vi "Input Multiplexer to FFT (2 inputs)_I16.vi"(7 "Reset?":bool, 8 "Input Data Valid Array":bool[](array[boolean])=[FALSE, FALSE], 11 "Input Data":fxp<+/-,16,2>[](array[numeric])=[0.0, 0.0]) -> (0 "Output Data Valid Array":bool[](array[boolean]), 3 "Interchanged Data":fxp<+/-,16,2>[](array[numeric]) format="%.15g")   [LabVIEW 2011]
uses:
  <userlib>/FPGA Library/Code Development/Signal Processing/Input Multiplexer to FFT/2 Input MUX/Input Index(Type) 2 inputs.ctl
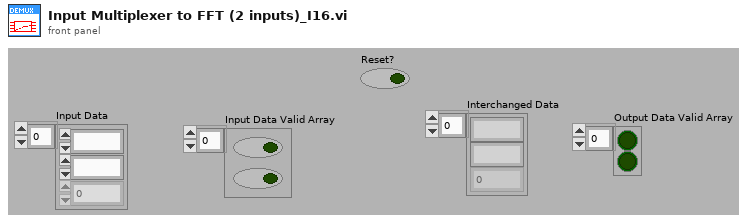
[diagram p1: front panel]
types:
  T1 = typedef "Input Index(Type) 2 inputs.ctl" = fxp<+,1,1>
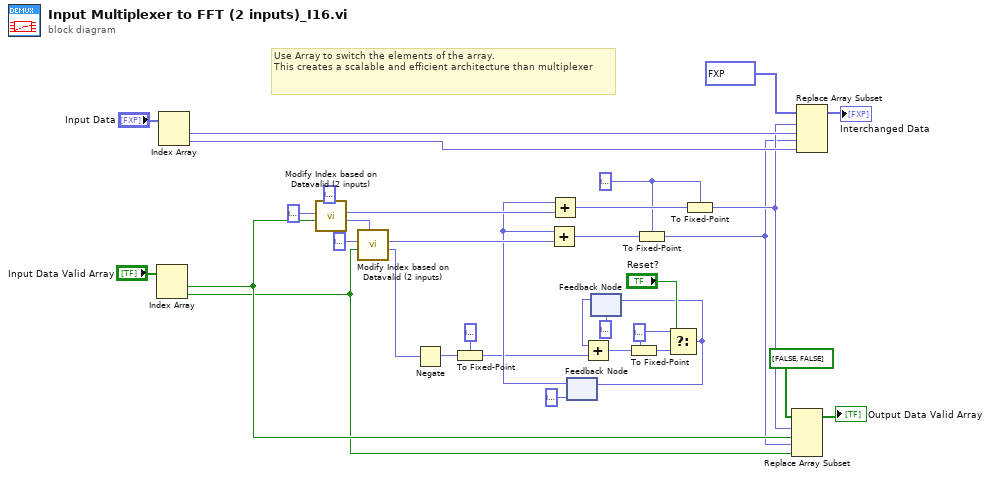
[diagram p0: block diagram]
diagram:
  w14 = T1 0.0
  w6 = T1 0.0 ("Actual Index")
  # "Use Array to switch the elements of the array. \nThis creates a scalable and efficient architecture than multiplexer"
  n1 = Index Array(array="Input Data Valid Array") -> (element #1=w30:bool, element #2=w29:bool)  [unwired: 2 in]
  n2 = Index Array(array="Input Data") -> (element #1=w21:fxp<+/-,16,2>, element #2=w20:fxp<+/-,16,2>)  [unwired: 2 in]
  n3 = call <userlib>:"Modify Index based on Datavalid (2 inputs).vi"("previous counter val"=T1 0.0, "cuurent index data valid?"=w30, "Actual Index"=T1 0.0) -> ("Next Counter Val"=w31:T1, "Modified Index"=w28:T1)  [unwired: 7 in]
  n4 = call <userlib>:"Modify Index based on Datavalid (2 inputs).vi"("previous counter val"=w31, "cuurent index data valid?"=w29, "Actual Index"=T1 1.0) -> ("Next Counter Val"=w3:T1, "Modified Index"=w26:T1)  [unwired: 7 in]
  n5 = Negate(x=w3) -> (-x=w10:fxp<+/-,1,1>)
  n6 = To Fixed-Point(fixed-point type=T1 0.0 ("Current Index Sum"), number=w10) -> (fixed-point=w9:T1)
  n7 = feedback #1(T1 0.0 ("Current Index Sum")) -> (w24:T1)
  n8 = Add(x=w24, y=w26) -> (x+y=w16:fxp<+,2,2>)
  n9 = Add(x=w24, y=w28) -> (x+y=w27:fxp<+,2,2>)
  n10 = feedback #2(T1 0.0) -> (w23:T1)
  n11 = Add(x=w23, y=w9) -> (x+y=w15:fxp<+,2,2>)
  n12 = To Fixed-Point(fixed-point type=w6, number=w15) -> (fixed-point=w7:T1)
  n13 = To Fixed-Point(fixed-point type=w14, number=w16) -> (fixed-point=w11:T1)
  n14 = Select(t=w6, s="Reset?", f=w7) -> (s? t:f=w4:T1)
  n15 = feedback-in #1(w4) -> ()
  n16 = feedback-in #2(w4) -> ()
  n17 = To Fixed-Point(fixed-point type=w14, number=w27) -> (fixed-point=w12:T1)
  n18 = Replace Array Subset(array=bool[] [FALSE, FALSE] ("appended array"), new element #1=w30, index #1=w12, new element #2=w29, index #2=w11) -> (→"Output Data Valid Array":bool[])
  n19 = Replace Array Subset(array=fxp<+/-,16,2>[] [0.0, 0.0], new element #1=w21, index #1=w12, new element #2=w20, index #2=w11) -> (→"Interchanged Data":fxp<+/-,16,2>[])
